vi "get array from reference.vi"(8 "error in (no error)":errorcluster, 11 "Autofocus in":refnum<class "Autofocus.lvclass">) -> (0 "error out":errorcluster, 3 "Autofocus out":refnum<class "Autofocus.lvclass">)   [LabVIEW 2012, in "Autofocus.lvclass"]
uses:
  Autofocus.lvclass
  Autofocus.lvclass/Autofocus.ctl
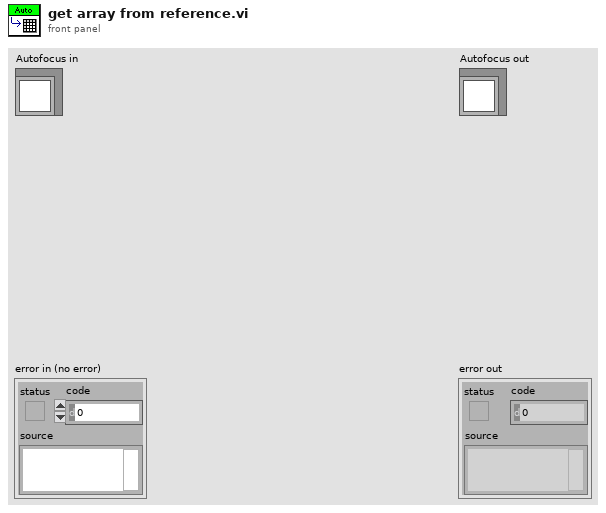
[diagram p1: front panel]
types:
  T1 = typedef "IMAQ Image.ctl" = refnum<image>
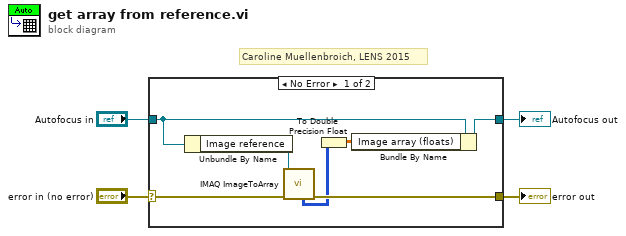
[diagram p0: block diagram]
diagram:
  # "Caroline Muellenbroich, LENS 2015"
  n1 = case shown="No Error" "error in (no error)" {
    selector: "error in (no error)" -> [w10 w13]
    tunnel: [w9 w13] -> w3
    tunnel: [w7 w12] -> w1
    tunnel: "Autofocus in" -> [w8 w12]
    frame No Error {
      n2 = Unbundle By Name(w8) -> ("Image reference"=w11:T1)
      n3 = call "IMAQ ImageToArray"("error in (no error)"=w10, "Image"=w11) -> ("Image Pixels (U16)"=w6:u16[][], "error out"=w9:errorcluster)  [unwired: 2 in, 3 out]
      n4 = To Double Precision Float(number=w6) -> (double precision float=w5:dbl[][])
      n5 = Bundle By Name(cluster=w8, "Image array (floats)"=w5) -> (w7:refnum<class "Autofocus.lvclass">)
    }
    frame Error {
    }
  }
  "error out" <- w3
  "Autofocus out" <- w1
